vi "LVLM - Slave Send and Receive.vi"   [LabVIEW 2010]
uses:
  <vilib>/NXT/Block Support/HWPage.SensorType.ctl
  <vilib>/NXT/Block Support/HWPage.SensorMode.ctl
  <vilib>/NXT/Block Support/NXT_InputPort.ctl
  <vilib>/NXT/Dual Mode Library/Sensors/i2c_sensors_big.vi
  <vilib>/NXT/Dual Mode Library/Display/drawText.vi
types:
  T1 = typedef "NXT_InputPort.ctl" = u8
  T2 = typedef "HWPage.SensorType.ctl" = u8
  T3 = typedef "HWPage.SensorMode.ctl" = u8
  T4 = typedef "LVHSConnector.ctl" = cluster{"Hardware":string, "Flattened String":string}
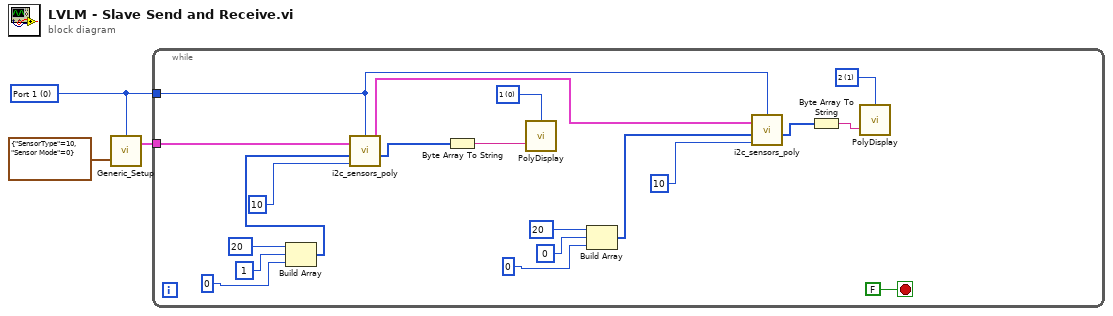
[diagram p0: block diagram]
diagram:
  w1 = T1 0 items=["Port 1", "Port 2", "Port 3", "Port 4"] ("Port")
  n1 = call <vilib>:"Generic_Setup.vi"("Sensor Setup"=cluster{"SensorType":T2, "Sensor Mode":T3} {"SensorType"=10, "Sensor Mode"=0}, "Port"=w1) -> ("NXT"=w2:T4)  [unwired: 1 in, 1 out]
  n2 = while {
    tunnel: w2 -> [w22]
    tunnel: w1 -> [w4]
    stop <- FALSE stop-if-true
    w6 = i16 1 items=["1", "2", "3", "4", "5", "6", "7", "8"] ("Line")
    w14 = i16 0 items=["1", "2", "3", "4", "5", "6", "7", "8"] ("Line")
    n3 = Build Array(u8 20, 1, 0 ("element")) -> (w18:i32[])
    n4 = call-poly <vilib>:"i2c_sensors_poly.vi"("Return Length"=u8 10, "Bytes to Write"=w18, "NXT"=w22, "Port"=w4) -> ("Bytes read"=w17:u8[], "NXT"=w5:T4)  [unwired: 1 in, 1 out]
    n5 = Byte Array To String(unsigned byte array=w17) -> (string=w16:string)
    n6 = call-poly <vilib>:"PolyDisplay.vi"("Text"=w16, "Line"=w14) -> ()  [unwired: 2 in, 1 out]
    n7 = Build Array(u8 20, 0, 0 ("element")) -> (w10:i32[])
    n8 = call-poly <vilib>:"i2c_sensors_poly.vi"("Return Length"=u8 10, "Bytes to Write"=w10, "NXT"=w5, "Port"=w4) -> ("Bytes read"=w9:u8[])  [unwired: 1 in, 2 out]
    n9 = Byte Array To String(unsigned byte array=w9) -> (string=w8:string)
    n10 = call-poly <vilib>:"PolyDisplay.vi"("Text"=w8, "Line"=w6) -> ()  [unwired: 2 in, 1 out]
  }
